vi "Configure Frequency Dependent Table.vi"(6 "Operation (0: Active Existing Table)":i32(ring) items=["Active Existing Table", "Define Frequency Array", "Define Gain Array", "Rename Existing Table", "Clear Existing Table"], 7 "New Table Name (\"MyTable\")":string="MyTable", 8 "error in (no error)":errorcluster, 9 "Table Name (\"CUSTOM_A\")":string="CUSTOM_A", 10 "Table Data":i32[](array[numeric]), 11 "VISA resource name":refnum<visa-resource-name>) -> (0 "error out":errorcluster, 3 "VISA resource name out":refnum<visa-resource-name>)   [LabVIEW 2018, in "Agilent U2000 Series.lvlib"]
doc: "Operates instrument for frequency-dependent table functionality. Includes:Defines, Actives, renames or clears specified frequency-dependent table.\n\nNote:\nStored tables remain in the U2000 Series power sensor memory during power down. The U2000 Series power sensor is capable of storing 10 frequency-dependent offset tables of 80 frequency points each."
uses:
  Agilent U2000 Series.lvlib
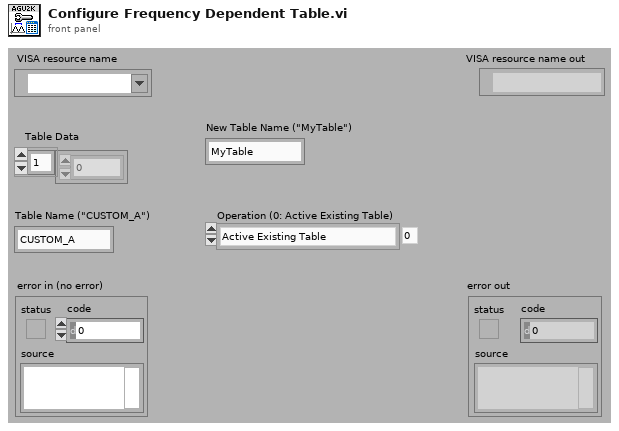
[diagram p1: front panel]
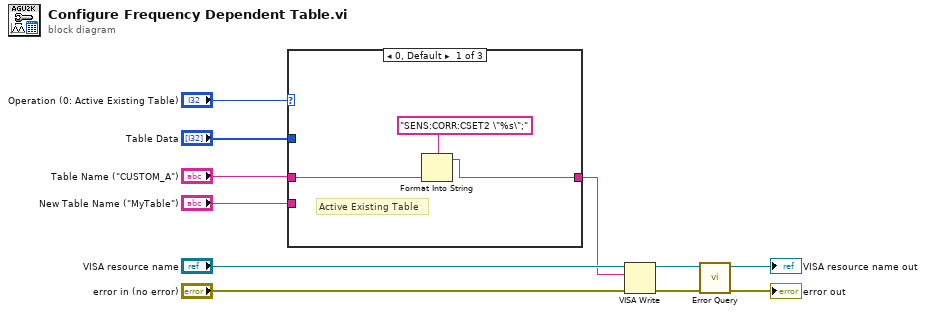
[diagram p0: block diagram]
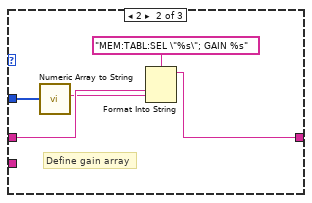
[diagram p2: hidden frame]
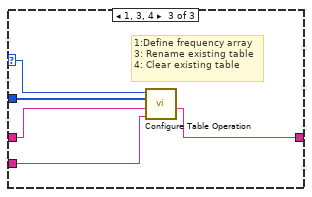
[diagram p3: hidden frame]
diagram:
  n1 = case shown="0, Default" "Operation (0: Active Existing Table)" {
    selector: "Operation (0: Active Existing Table)" -> [_ _ w24]
    tunnel: [w12 w18 w20] -> w6
    tunnel: "Table Name (\"CUSTOM_A\")" -> [w14 w17 w22]
    tunnel: "New Table Name (\"MyTable\")" -> [_ _ w21]
    tunnel: "Table Data" -> [_ w16 w23]
    frame 0, Default {
      # "Active Existing Table"
      n2 = Format Into String(format string="SENS:CORR:CSET2 \"%s\";", w14) -> (resulting string=w12:string)  [unwired: 2 in, 1 out]
    }
    frame 2 {
      # "Define gain array"
      n3 = call "Numeric Array to String.vi"("List Data"=w16) -> ("Result String"=w15:string)  [unwired: 10 out]
      n4 = Format Into String(format string="MEM:TABL:SEL \"%s\"; GAIN %s", w17, w15) -> (resulting string=w18:string)  [unwired: 2 in, 1 out]
    }
    frame 1, 3, 4 {
      # "1:Define frequency array\n3: Rename existing table\n4: Clear existing table"
      n5 = call "Configure Table Operation.vi"("New Table Name (\"MyTable\")"=w21, "Table Name (\"DEFAULT\")"=w22, "Table Data"=w23, "Operation (1: Define Frequency Array)"=w24) -> ("ResultString"=w20:string)  [unwired: 7 in]
    }
  }
  n6 = VISA Write(VISA resource name="VISA resource name", write buffer=w6, error in (no error)="error in (no error)") -> (VISA resource name out=w5:refnum<visa-resource-name>, error out=w4:errorcluster)  [unwired: 1 out]
  n7 = call "Error Query.vi"("error in (no error)"=w4, "VISA resource name"=w5) -> ("error out"=→"error out":errorcluster, "VISA resource name out"=→"VISA resource name out":refnum<visa-resource-name>)  [unwired: 8 out]
